vi "V50 Report Threat (SubVI).vi"(0 "NI_report in":refnum<class "NI_report.lvclass">, 5 "SampleID":string, 11 "error in (no error)":errorcluster) -> (4 "NI_report out":refnum<class "NI_report.lvclass">, 15 "error out":errorcluster)   [LabVIEW 2015]
uses:
  <vilib>/Utility/NIReport.llb/NI_report.lvclass
panel:
  out "appended array":string[][](array[string])
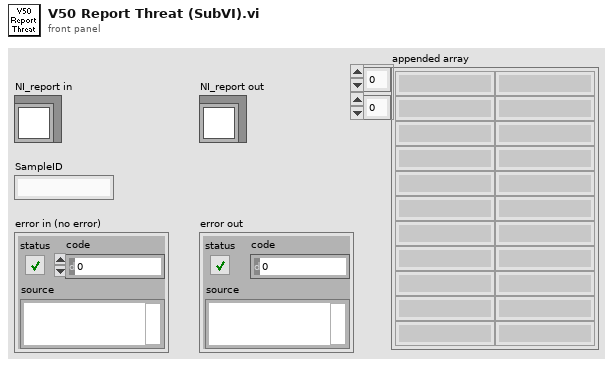
[diagram p1: front panel]
types:
  T1 = cluster{"position (excel)":cluster{"row":i32, "column":i32}, "name (excel)":string, "bookmark (word)":string}
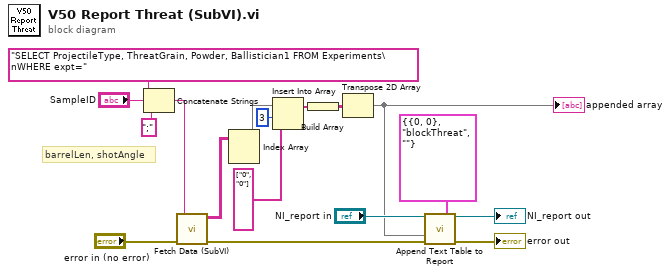
[diagram p0: block diagram]
diagram:
  # "barrelLen, shotAngle"
  n1 = Concatenate Strings("SELECT ProjectileType, ThreatGrain, Powder, Ballistician1 FROM Experiments\nWHERE expt=" ("query string"), "SampleID", ";" ("string")) -> (w14:string)
  n2 = call "Fetch Data (SubVI).vi"("error IN"="error in (no error)", "query string"=w14) -> ("error OUT"=w8:errorcluster, "recordset data"=w6:string[][])  [unwired: 4 out]
  n3 = Index Array(array=w6) -> (element=w3:string[])  [unwired: 2 in]
  n4 = Insert Into Array(array=w3, index=3 ("index (row)"), new element=string[] ["0", "0"] ("new element/subarray")) -> (w1:string[])
  n5 = Build Array(w1) -> (w2:string[][])
  n6 = Transpose 2D Array(2D array=w2) -> (transposed array=w7:string[][])
  "appended array" <- w7
  n7 = call-dynamic "Append Text Table to Report.vi"("report in"="NI_report in", "MS Office parameters"=T1 {"position (excel)"={"row"=0, "column"=0}, "name (excel)"="blockThreat", "bookmark (word)"=""}, "text data"=w7, "error in (no error)"=w8) -> ("report out"=→"NI_report out":refnum<class "NI_report.lvclass">, "error out"=→"error out":errorcluster)  [unwired: 8 in, 2 out]
